vi "Create DVR.vi"(8 "error in (no error)":errorcluster, 11 "data value":dbl) -> (0 "error out":errorcluster, 3 "data value reference":refnum<data-value>)   [LabVIEW 2015]
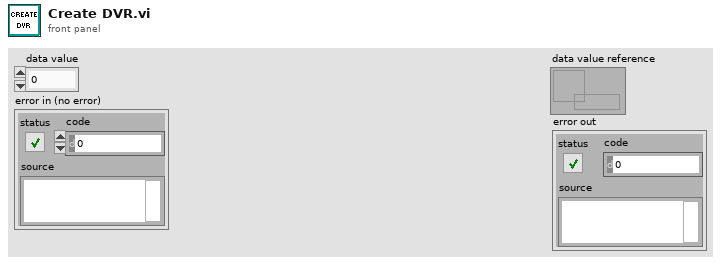
[diagram p1: front panel]
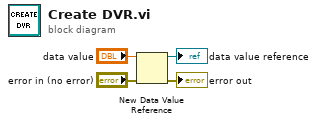
[diagram p0: block diagram]
diagram:
  n1 = New Data Value Reference(data value="data value", error in="error in (no error)") -> (data value reference=→"data value reference":refnum<data-value>, error out=→"error out":errorcluster)
